vi "Screen_ShowHseAbout.vi"(8 "error in":errorcluster) -> (0 "error out":errorcluster)   [LabVIEW 2020, in "hse-ui.lvlib"]
doc: "____\nHAMPEL SOFTWARE ENGINEERING v3.8.0 (2023-12-18 14:41)"
uses:
  hse-ui.lvlib
  HSE_AboutScreen.vi
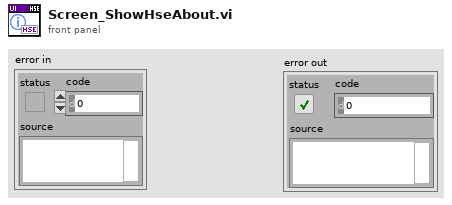
[diagram p1: front panel]
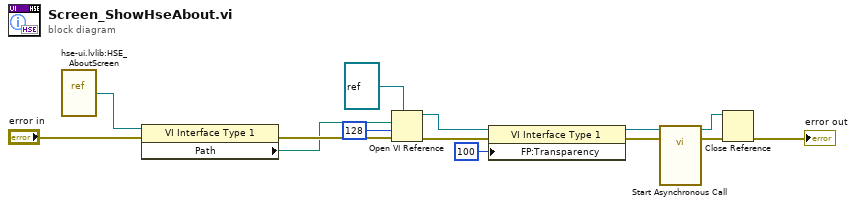
[diagram p0: block diagram]
diagram:
  n1 = vi-ref "hse-ui.lvlib:HSE_AboutScreen.vi"() -> (w9:refnum<vi>)
  n2 = property class="VI Interface Type 1"(reference=w9, error in="error in") -> (error out=w7:errorcluster, "Path"=w6:path)  [unwired: 1 out]
  n3 = Open VI Reference(type specifier VI Refnum (for type only)=refnum<vi> refnum, vi path=w6, options=128, error in (no error)=w7) -> (vi reference=w3:refnum<vi>, error out=w4:errorcluster)  [unwired: 2 in]
  n4 = property class="VI Interface Type 1"(reference=w3, error in=w4, "FP:Transparency"=u8 100 ("Front Panel Window:Transparency")) -> (reference out=w1:refnum<vi>, error out=w2:errorcluster)
  n5 = call-by-ref "Start Asynchronous Call"(reference=w1, error in=w2) -> (reference out=w12:refnum<vi>, error out=w11:errorcluster)  [unwired: 12 in]
  n6 = Close Reference(reference=w12, error in (no error)=w11) -> (error out=→"error out":errorcluster)
